vi "BalanceMotorControl2.vi"(8 "Number of Motors":i16, 9 "PID Gains":T1(array[cluster]) {"derivative time (Td, min)" format="%.3f"; "integral time (Ti, min)" format="%.3f"; "proportional gain (Kc)" format="%.3f"}, 11 "Gx, Gy, wz":dbl[](array[numeric])) -> (3 "Motor Controls":dbl[](array[numeric]))   [LabVIEW 2017]
uses:
  <vilib>/addons/control/pid/pid.llb/PID (DBL Array).vi
  <vilib>/addons/control/pid/NI_PID_pid.lvlib
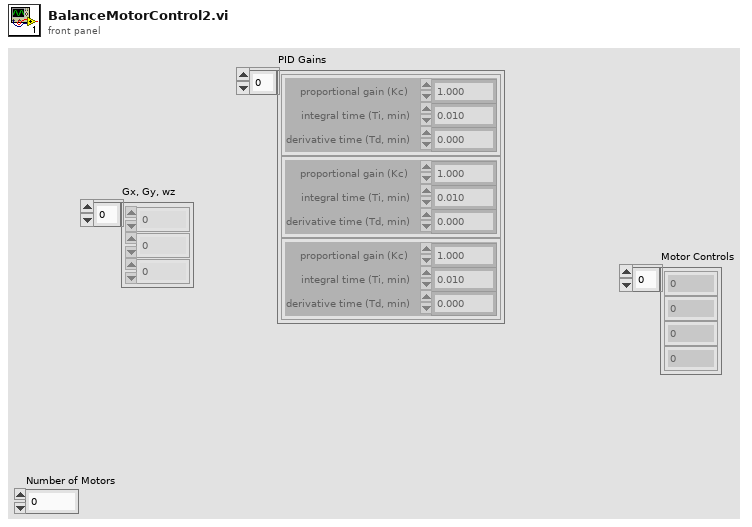
[diagram p1: front panel]
types:
  T1 = cluster{"proportional gain (Kc)":dbl, "integral time (Ti, min)":dbl, "derivative time (Td, min)":dbl}[]
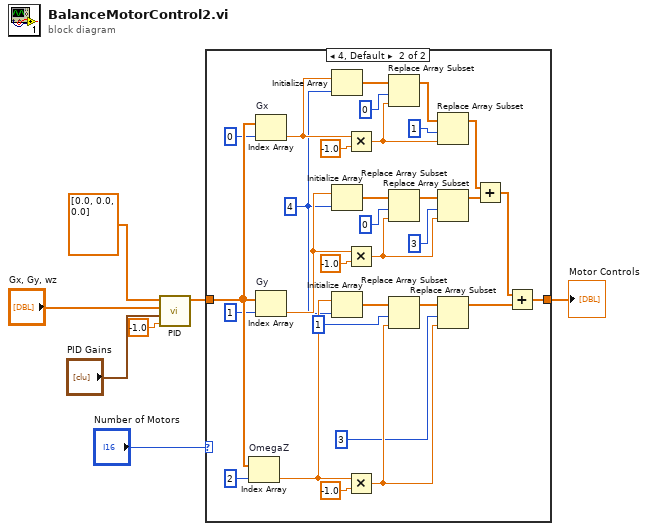
[diagram p0: block diagram]
diagram:
  n1 = call-poly <vilib>:"PID.vi"("dt (s)"=-1.0, "PID gains"="PID Gains", "process variable"="Gx, Gy, wz", "setpoint"=dbl[] [0.0, 0.0, 0.0]) -> ("output"=w4:dbl[])  [unwired: 6 in, 1 out]
  n2 = case shown="4, Default" "Number of Motors" {
    tunnel: w4 -> [w8 w39]
    tunnel: [w8 w19] -> w3
    frame 6 {
    }
    frame 4, Default {
      w12 = 4 ("dimension size")
      n3 = Index Array "OmegaZ"(array=w39, index=2) -> (element=w35:dbl)
      n4 = Index Array "Gx"(array=w39, index=0) -> (element=w38:dbl)
      n5 = Index Array "Gy"(array=w39, index=1) -> (element=w36:dbl)
      n6 = Initialize Array(w38, w12) -> (w32:dbl[])
      n7 = Initialize Array(w36, w12) -> (w29:dbl[])
      n8 = Initialize Array(w35, w12) -> (w26:dbl[])
      n9 = Multiply(x=w38, y=-1.0) -> (x*y=w30:dbl)
      n10 = Multiply(x=w36, y=-1.0) -> (x*y=w27:dbl)
      n11 = Multiply(x=w35, y=-1.0) -> (x*y=w24:dbl)
      n12 = Replace Array Subset(array=w32, new element=w30, index=0) -> (w31:dbl[])
      n13 = Replace Array Subset(array=w29, new element=w27, index=0) -> (w28:dbl[])
      n14 = Replace Array Subset(array=w26, new element=w24, index=i16 1 ("Motors 1 or 3")) -> (w25:dbl[])
      n15 = Replace Array Subset(array=w31, new element=w30, index=1) -> (w23:dbl[])
      n16 = Replace Array Subset(array=w28, new element=w27, index=3) -> (w22:dbl[])
      n17 = Replace Array Subset(array=w25, new element=w24, index=i16 3 ("Motors 2 or 4")) -> (w21:dbl[])
      n18 = Add(x=w23, y=w22) -> (x+y=w20:dbl[])
      n19 = Add(x=w20, y=w21) -> (x+y=w19:dbl[])
    }
  }
  "Motor Controls" <- w3
